vi "CRYCalc standard deviation.vi"(6 "Work in":u16, 7 "Step Setup VI No":i32, 8 "Statistic Run Number":i32, 10 "+/-Adjust(Deviation)":i32, 11 "Data in":T1 {"Z data" items=["dB", "Lin"]; "X data" items=["dB", "Lin"]; "Y data" items=["dB", "Lin"]; "Z dB ref" format="%.1f"; "Z axis" items=["Log", "Lin"]; "X dB ref" format="%.1f"; "X axis" items=["Log", "Lin"]; "Y axis" items=["Log", "Lin"]; "Y dB ref" format="%.1f"; "Curve"."z" format="%.2f"; "Curve"."y" format="%.2f"; "Curve"."x" format="%.2f"}) -> (1 "Absolute StanDev Out":T1 {"Z data" items=["dB", "Lin"]; "X data" items=["dB", "Lin"]; "Y data" items=["dB", "Lin"]; "Z dB ref" format="%.1f"; "Z axis" items=["Log", "Lin"]; "X dB ref" format="%.1f"; "X axis" items=["Log", "Lin"]; "Y axis" items=["Log", "Lin"]; "Y dB ref" format="%.1f"; "Curve"."z" format="%.2f"; "Curve"."y" format="%.2f"; "Curve"."x" format="%.2f"}, 2 "Mean Out":T1 {"Z data" items=["dB", "Lin"]; "X data" items=["dB", "Lin"]; "Y data" items=["dB", "Lin"]; "Z dB ref" format="%.1f"; "Z axis" items=["Log", "Lin"]; "X dB ref" format="%.1f"; "X axis" items=["Log", "Lin"]; "Y axis" items=["Log", "Lin"]; "Y dB ref" format="%.1f"; "Curve"."z" format="%.2f"; "Curve"."y" format="%.2f"; "Curve"."x" format="%.2f"}, 3 "Standard dev Out":T1 {"Z data" items=["dB", "Lin"]; "X data" items=["dB", "Lin"]; "Y data" items=["dB", "Lin"]; "Z dB ref" format="%.1f"; "Z axis" items=["Log", "Lin"]; "X dB ref" format="%.1f"; "X axis" items=["Log", "Lin"]; "Y axis" items=["Log", "Lin"]; "Y dB ref" format="%.1f"; "Curve"."z" format="%.2f"; "Curve"."y" format="%.2f"; "Curve"."x" format="%.2f"})   [LabVIEW 2013]
uses:
  Typedef Control/CRYData Cluster Array.ctl
  Typedef Control/CRYData Cluster.ctl
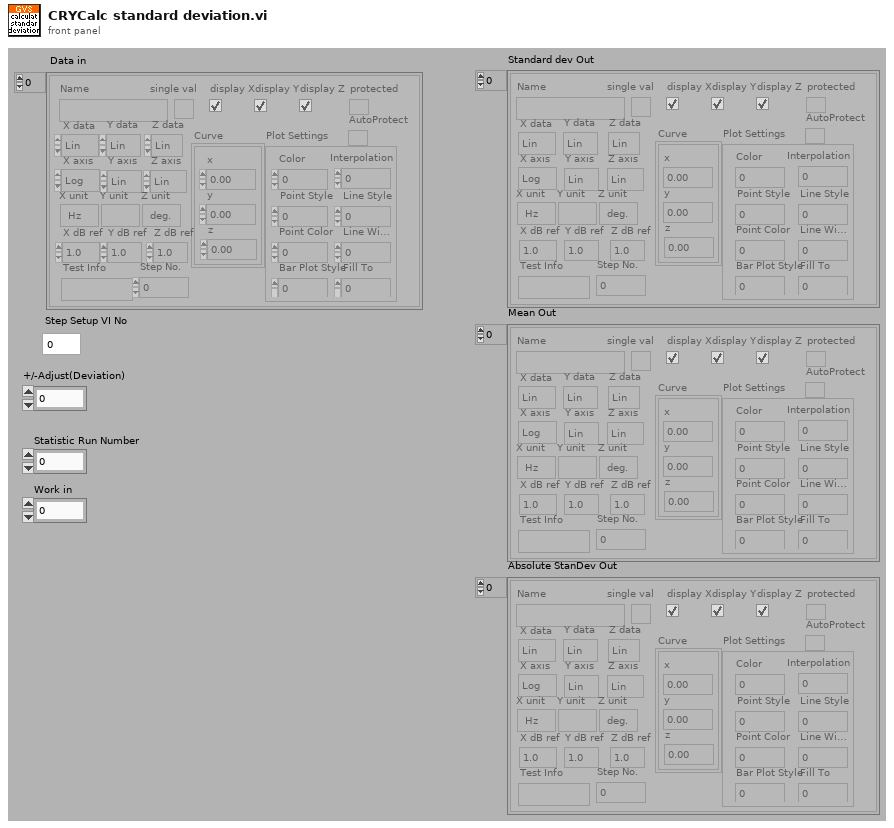
[diagram p1: front panel]
types:
  T1 = typedef "CRYData Cluster Array.ctl" = T2[]
  T2 = typedef "CRYData Cluster.ctl" = cluster{"Name":string, "Curve":cluster{"x":dbl, "y":dbl, "z":dbl}[], "X data":u16, "Y data":u16, "Z data":u16, "X axis":u16, "Y axis":u16, "Z axis":u16, "X unit":string, "Y unit":string, "Z unit":string, "X dB ref":dbl, "Y dB ref":dbl, "Z dB ref":dbl, "single val":bool, "protected":bool, "display X":bool, "display Y":bool, "display Z":bool, "Test Info":string, "Step No.":i32, "Plot Settings":cluster{"Color":u32, "Interpolation":u8, "Point Style":u8, "Line Style":u8, "Point Color":u32, "Line Width":u8, "Bar Plot Style":u8, "Fill To":i16}, "AutoProtect":bool}
  T3 = enum32{"English", "Chinese", "Korean", "Japanese", "Russian", "Chinese traditional"}
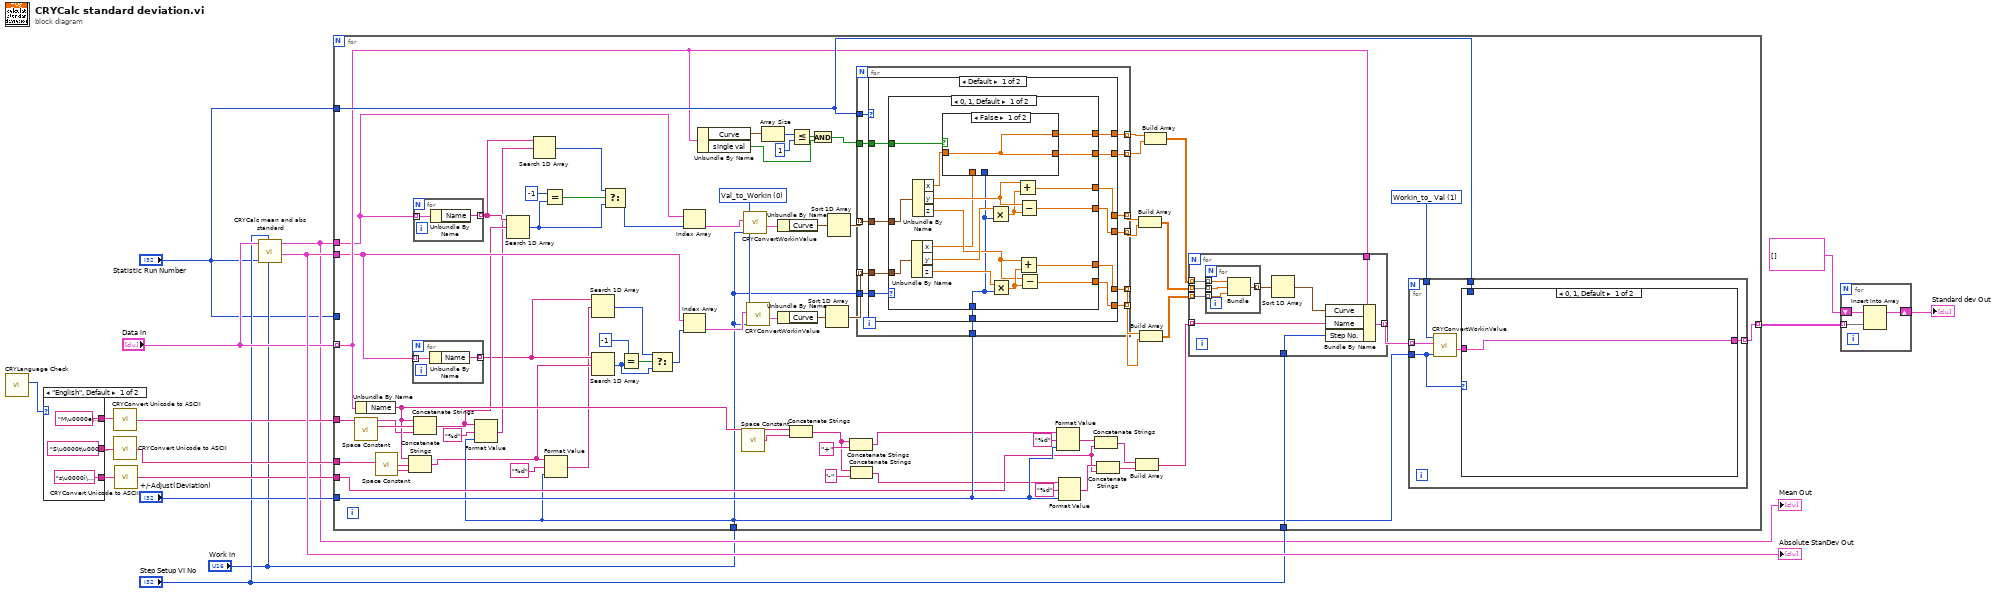
[diagram p0: block diagram]
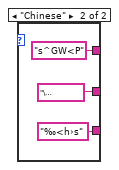
[diagram p2: hidden frame]
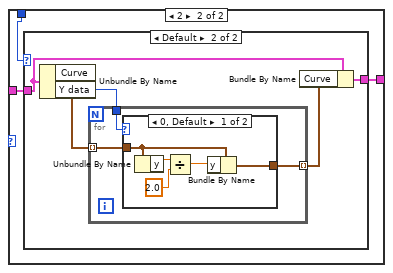
[diagram p3: hidden frame]
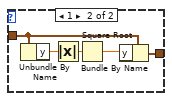
[diagram p5: hidden frame]
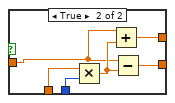
[diagram p6: hidden frame]
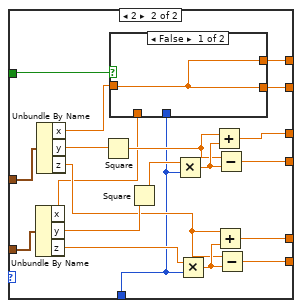
[diagram p7: hidden frame]
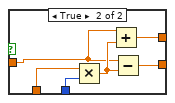
[diagram p8: hidden frame]
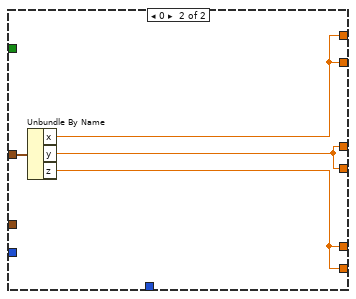
[diagram p9: hidden frame]
diagram:
  n1 = call "CRYLanguage Check.vi"() -> ("Language"=w10:T3)  [unwired: 10 in, 1 out]
  n2 = case shown="\"English\", Default" w10 {
    tunnel: ["M\u0000e\u0000a\u0000n\u0000" ("format string") "s^GW<P" ("format string")] -> w11
    tunnel: ["S\u0000t\u0000d\u0000 \u0000D\u0000e\u0000v\u0000" ("format string") "\u0007hÆQî]" ("format string")] -> w9
    tunnel: ["s\u0000i\u0000g\u0000m\u0000a\u0000" "‰<h›s" ("format string")] -> w8
    frame "English", Default {
    }
    frame "Chinese" {
    }
  }
  n3 = call "CRYConvert Unicode to ASCII.vi"("Unicode"=w11) -> ("ASCII"=w7:string)  [unwired: 4 in]
  n4 = call "CRYConvert Unicode to ASCII.vi"("Unicode"=w9) -> ("ASCII"=w6:string)  [unwired: 4 in]
  n5 = call "CRYConvert Unicode to ASCII.vi"("Unicode"=w8) -> ("ASCII"=w5:string)  [unwired: 4 in]
  n6 = call "CRYCalc mean and abs standard.vi"("Work in"="Work in", "Step Setup VI No"="Step Setup VI No", "Statistic Run Number"="Statistic Run Number", "Data in"="Data in") -> ("Absolute StanDev Out"=w15:T1, "Mean Out"=w3:T1)  [unwired: 5 in, 1 out]
  "Mean Out" <- w3
  "Absolute StanDev Out" <- w15
  n7 = for {
    tunnel: w3 -> [w30]
    tunnel: w15 -> [w40]
    tunnel: "Data in" -> [w43] mode=indexing
    tunnel: "+/-Adjust(Deviation)" -> [w80]
    tunnel: [w57] -> w12 mode=indexing
    tunnel: "Step Setup VI No" -> [w76]
    tunnel: w7 -> [w75]
    tunnel: w6 -> [w74]
    tunnel: w5 -> [w66]
    tunnel: "Work in" -> [w42]
    tunnel: "Statistic Run Number" -> [w44]
    tunnel: "Statistic Run Number" -> [_]
    w56 = u16 1 items=["Val_to_Workin", "Workin_to_ Val"] ("Type")
    w59 = u16 0 items=["Val_to_Workin", "Workin_to_ Val"] ("Type")
    n8 = call <vilib>:"Space Constant.vi"() -> ("String"=w94:string)
    n9 = Unbundle By Name(w43) -> ("Name"=w81:string)
    n10 = call <vilib>:"Space Constant.vi"() -> ("String"=w93:string)
    n11 = Concatenate Strings(w81, w93, w74) -> (w26:string)
    n12 = for {
      tunnel: w40 -> [w98] mode=indexing
      tunnel: [w97] -> w25 mode=indexing
      n13 = Unbundle By Name(w98) -> ("Name"=w97:string)
    }
    n14 = for {
      tunnel: w30 -> [w96] mode=indexing
      tunnel: [w95] -> w28 mode=indexing
      n15 = Unbundle By Name(w96) -> ("Name"=w95:string)
    }
    n16 = Concatenate Strings(w81, w94, w75) -> (w29:string)
    n17 = Format Value(string ("")=w29, format string="%d", value (0)=w42) -> (output string=w27:string)
    n18 = Search 1D Array(1D array=w28, element=w29) -> (index of element=w31:i32)  [unwired: 1 in]
    n19 = Search 1D Array(1D array=w28, element=w27) -> (index of element=w34:i32)  [unwired: 1 in]
    n20 = Equal?(x=-1 ("y"), y=w31) -> (x = y?=w33:bool)
    n21 = Format Value(string ("")=w26, format string="%d", value (0)=w42) -> (output string=w24:string)
    n22 = Search 1D Array(1D array=w25, element=w24) -> (index of element=w39:i32)  [unwired: 1 in]
    n23 = Search 1D Array(1D array=w25, element=w26) -> (index of element=w37:i32)  [unwired: 1 in]
    n24 = Select(t=w34, s=w33, f=w31) -> (s? t:f=w32:i32)
    n25 = Equal?(x=-1 ("y"), y=w37) -> (x = y?=w41:bool)
    n26 = Select(t=w39, s=w41, f=w37) -> (s? t:f=w36:i32)
    n27 = Index Array(array=w30, index=w32) -> (element=w63:T2)
    n28 = Index Array(array=w40, index=w36) -> (element=w61:T2)
    n29 = Unbundle By Name(w43) -> ("Curve"=w51:cluster{"x":dbl, "y":dbl, "z":dbl}[], "single val"=w55:bool)
    n30 = call <vilib>:"Space Constant.vi"() -> ("String"=w84:string)
    n31 = call "CRYConvertWorkinValue.vi"("Work in"=w42, "In"=w63, "Type"=w59) -> ("Out"=w62:T2)  [unwired: 8 in]
    n32 = call "CRYConvertWorkinValue.vi"("Work in"=w42, "In"=w61, "Type"=w59) -> ("Out"=w60:T2)  [unwired: 8 in]
    n33 = Array Size(array=w51) -> (size(s)=w52:i32)
    n34 = Unbundle By Name(w62) -> ("Curve"=w92:cluster{"x":dbl, "y":dbl, "z":dbl}[])
    n35 = Unbundle By Name(w60) -> ("Curve"=w91:cluster{"x":dbl, "y":dbl, "z":dbl}[])
    n36 = Concatenate Strings(w81, w84) -> (w72:string)
    n37 = Less Or Equal?(x=w52, y=1) -> (x <= y?=w54:bool)
    n38 = And(x=w54, y=w55) -> (x .and. y?=w50:bool)
    n39 = Sort 1D Array(array=w91) -> (sorted array=w77:cluster{"x":dbl, "y":dbl, "z":dbl}[])
    n40 = Sort 1D Array(array=w92) -> (sorted array=w78:cluster{"x":dbl, "y":dbl, "z":dbl}[])
    n41 = Concatenate Strings(w72, "+" ("format string")) -> (w65:string)
    n42 = Concatenate Strings(w72, "-" ("format string")) -> (w64:string)
    n43 = for {
      tunnel: [w139] -> w90 mode=indexing
      tunnel: [w138] -> w89 mode=indexing
      tunnel: [w137] -> w88 mode=indexing
      tunnel: [w136] -> w87 mode=indexing
      tunnel: w80 -> [w135]
      tunnel: w78 -> [w134] mode=indexing
      tunnel: w77 -> [w133] mode=indexing
      tunnel: w42 -> [w132]
      tunnel: w44 -> [w131]
      tunnel: w50 -> [w130]
      tunnel: [w129] -> w48 mode=indexing
      tunnel: [w128] -> w49 mode=indexing
      n44 = case shown="Default" w131 {
        tunnel: [w150 w205] -> w139
        tunnel: [w149 w205] -> w138
        tunnel: [w148 w204] -> w137
        tunnel: [w147 w204] -> w136
        tunnel: w135 -> [w146 _]
        tunnel: w134 -> [w145 w206]
        tunnel: w133 -> [w144 _]
        tunnel: w132 -> [w143 _]
        tunnel: w130 -> [w142 _]
        tunnel: [w141 w203] -> w129
        tunnel: [w140 w203] -> w128
        frame Default {
          n45 = case shown="0, 1, Default" w143 {
            tunnel: [w167 w187] -> w150
            tunnel: [w166 w188] -> w149
            tunnel: [w165 w186] -> w148
            tunnel: [w164 w185] -> w147
            tunnel: w146 -> [w153 w178]
            tunnel: w145 -> [w161 w192]
            tunnel: w144 -> [w160 w191]
            tunnel: w142 -> [w156 w179]
            tunnel: [w154 w176] -> w141
            tunnel: [w151 w177] -> w140
            frame 0, 1, Default {
              n46 = Unbundle By Name(w160) -> ("x"=w152:dbl, "y"=w159:dbl, "z"=w158:dbl)
              n47 = Unbundle By Name(w161) -> ("x"=w155:dbl, "y"=w168:dbl, "z"=w157:dbl)
              n48 = case shown="False" w156 {
                tunnel: [w169 w171] -> w154
                tunnel: w155 -> [w169 w172]
                tunnel: w153 -> [_ w174]
                tunnel: w152 -> [_ w173]
                tunnel: [w169 w170] -> w151
                frame False {
                }
                frame True {
                  n49 = Multiply(x=w173, y=w174) -> (x*y=w175:dbl)
                  n50 = Add(x=w172, y=w175) -> (x+y=w170:dbl)
                  n51 = Subtract(x=w172, y=w175) -> (x-y=w171:dbl)
                }
              }
              n52 = Multiply(x=w159, y=w153) -> (x*y=w163:dbl)
              n53 = Multiply(x=w158, y=w153) -> (x*y=w162:dbl)
              n54 = Add(x=w168, y=w163) -> (x+y=w167:dbl)
              n55 = Add(x=w157, y=w162) -> (x+y=w165:dbl)
              n56 = Subtract(x=w168, y=w163) -> (x-y=w166:dbl)
              n57 = Subtract(x=w157, y=w162) -> (x-y=w164:dbl)
            }
            frame 2 {
              n58 = Unbundle By Name(w191) -> ("x"=w181:dbl, "y"=w184:dbl, "z"=w183:dbl)
              n59 = Unbundle By Name(w192) -> ("x"=w180:dbl, "y"=w195:dbl, "z"=w182:dbl)
              n60 = Square(x=w195) -> (x^2=w190:dbl)
              n61 = case shown="False" w179 {
                tunnel: [w196 w198] -> w176
                tunnel: w180 -> [w196 w199]
                tunnel: w178 -> [_ w201]
                tunnel: w181 -> [_ w200]
                tunnel: [w196 w197] -> w177
                frame False {
                }
                frame True {
                  n62 = Multiply(x=w200, y=w201) -> (x*y=w202:dbl)
                  n63 = Add(x=w199, y=w202) -> (x+y=w197:dbl)
                  n64 = Subtract(x=w199, y=w202) -> (x-y=w198:dbl)
                }
              }
              n65 = Square(x=w184) -> (x^2=w189:dbl)
              n66 = Multiply(x=w189, y=w178) -> (x*y=w194:dbl)
              n67 = Multiply(x=w183, y=w178) -> (x*y=w193:dbl)
              n68 = Add(x=w190, y=w194) -> (x+y=w187:dbl)
              n69 = Add(x=w182, y=w193) -> (x+y=w186:dbl)
              n70 = Subtract(x=w190, y=w194) -> (x-y=w188:dbl)
              n71 = Subtract(x=w182, y=w193) -> (x-y=w185:dbl)
            }
          }
        }
        frame 0 {
          n72 = Unbundle By Name(w206) -> ("x"=w203:dbl, "y"=w205:dbl, "z"=w204:dbl)
        }
      }
    }
    n73 = Format Value(string ("")=w65, format string="%d", value (0)=w80) -> (output string=w70:string)
    n74 = Format Value(string ("")=w64, format string="%d", value (0)=w80) -> (output string=w69:string)
    n75 = Concatenate Strings(w70, w66) -> (w68:string)
    n76 = Concatenate Strings(w69, w66) -> (w67:string)
    n77 = Build Array(w68, w67) -> (w79:string[])
    n78 = Build Array(w90, w89) -> (w86:dbl[][])
    n79 = Build Array(w88, w87) -> (w85:dbl[][])
    n80 = Build Array(w49, w48) -> (w47:dbl[][])
    n81 = for {
      tunnel: w47 -> [w215] mode=indexing
      tunnel: w85 -> [w214] mode=indexing
      tunnel: [w212] -> w58 mode=indexing
      tunnel: w79 -> [w209] mode=indexing
      tunnel: w86 -> [w211] mode=indexing
      tunnel: w43 -> [w210]
      tunnel: w76 -> [w207]
      n82 = for {
        tunnel: w211 -> [w218] mode=indexing
        tunnel: [w219] -> w213 mode=indexing
        tunnel: w215 -> [w217] mode=indexing
        tunnel: w214 -> [w216] mode=indexing
        n83 = Bundle("x"=w217, "y"=w218, "z"=w216) -> (w219:cluster{"x":dbl, "y":dbl, "z":dbl})  [unwired: 1 out]
      }
      n84 = Sort 1D Array(array=w213) -> (sorted array=w208:cluster{"x":dbl, "y":dbl, "z":dbl}[])
      n85 = Bundle By Name(cluster=w210, "Curve"=w208, "Name"=w209, "Step No."=w207) -> (w212:T2)
    }
    n86 = for {
      tunnel: w58 -> [w104] mode=indexing
      tunnel: [w101] -> w57 mode=indexing
      tunnel: w56 -> [w103]
      tunnel: w42 -> [w100]
      tunnel: w44 -> [w99]
      n87 = call "CRYConvertWorkinValue.vi"("Work in"=w100, "In"=w104, "Type"=w103) -> ("Out"=w102:T2)  [unwired: 8 in]
      n88 = case shown="0, 1, Default" w100 {
        tunnel: w102 -> [w105 w108]
        tunnel: [w105 w107] -> w101
        tunnel: w99 -> [_ w106]
        frame 0, 1, Default {
        }
        frame 2 {
          n89 = case shown="Default" w106 {
            tunnel: w108 -> [w109 w112]
            tunnel: [w109 w111] -> w107
            frame 0 {
            }
            frame Default {
              n90 = Unbundle By Name(w112) -> ("Curve"=w114:cluster{"x":dbl, "y":dbl, "z":dbl}[], "Y data"=w110:u16)
              n91 = for {
                tunnel: w114 -> [w117] mode=indexing
                tunnel: [w116] -> w113 mode=indexing
                tunnel: w110 -> [w115]
                n92 = case shown="0, Default" w115 {
                  tunnel: w117 -> [w121 w127]
                  tunnel: [w118 w126] -> w116
                  frame 0, Default {
                    n93 = Unbundle By Name(w121) -> ("y"=w122:dbl)
                    n94 = Divide(x=w122, y=2.0) -> (x/y=w120:dbl)
                    n95 = Bundle By Name(cluster=w121, "y"=w120) -> (w118:cluster{"x":dbl, "y":dbl, "z":dbl})
                  }
                  frame 1 {
                    n96 = Unbundle By Name(w127) -> ("y"=w125:dbl)
                    n97 = Absolute Value(x=w125) -> (abs(x)=w123:dbl)
                    n98 = Square Root(x=w123) -> (sqrt(x)=w124:dbl)
                    n99 = Bundle By Name(cluster=w127, "y"=w124) -> (w126:cluster{"x":dbl, "y":dbl, "z":dbl})
                  }
                }
              }
              n100 = Bundle By Name(cluster=w112, "Curve"=w113) -> (w111:T2)
            }
          }
        }
      }
    }
  }
  n101 = for {
    tunnel: w12 -> [w222] mode=indexing
    shift-right: [w220] -> w16
    shift-left: T1 [] ("Data in") -> [w221]
    n102 = Insert Into Array(array=w221, new element=w222) -> (w220:T1)  [unwired: 1 in]
  }
  "Standard dev Out" <- w16
